vi "AddObject.vi"(8 "error in (no error)":errorcluster, 9 "OjbectName":string, 11 "Object2Add":refnum<class>) -> (0 "error out":errorcluster, 3 "ObjectOut":refnum<class>)   [LabVIEW 2021, in "Application.lvclass"]
uses:
  Application.lvclass
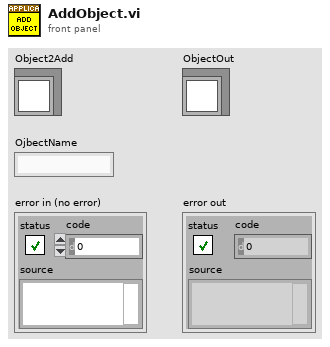
[diagram p1: front panel]
types:
  T1 = typedef "Application.lvclass/ObjectAttributes.ctl" = cluster{"Objects":variant, "BasePath":path, "Application":refnum<class "Application.lvclass">}
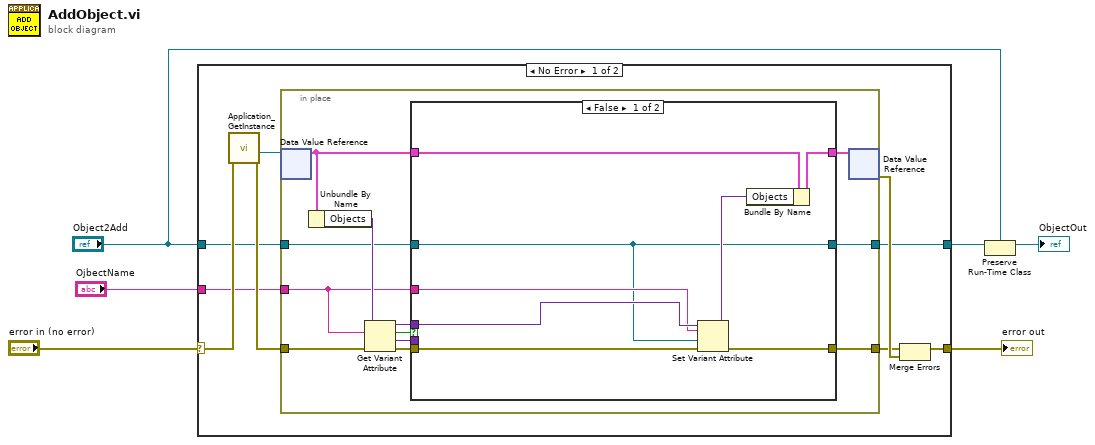
[diagram p0: block diagram]
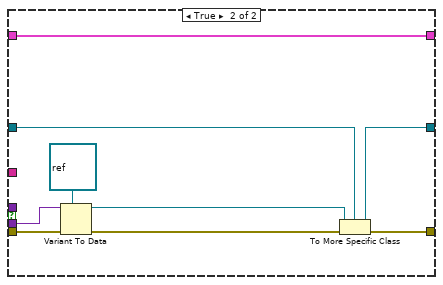
[diagram p2: hidden frame]
diagram:
  n1 = case shown="No Error" "error in (no error)" {
    selector: "error in (no error)" -> [w14 w45]
    tunnel: [w15 w45] -> w1
    tunnel: "OjbectName" -> [w10 _]
    tunnel: "Object2Add" -> [w9 _]
    tunnel: [w7 _] -> w5
    frame No Error {
      n2 = call "Application_GetInstance.vi"("error in"=w14) -> ("error out"=w11:errorcluster, "DVRRefOut"=w13:refnum<data-value>)  [unwired: 6 in, 3 out]
      n3 = in-place {
        in-place-border: w11 -> [w25]
        in-place-border: w10 -> [w17]
        in-place-border: w9 -> [w20]
        in-place-border: [w19] -> w8
        in-place-border: [w18] -> w7
        n4 = in-place-dvr #1(w13) -> (w26:T1)  [unwired: 1 out]
        n5 = Unbundle By Name(w26) -> ("Objects"=w24:variant)
        n6 = Get Variant Attribute(Variant=w24, name=w17, error in=w25) -> (duplicate Variant=w21:variant, found=w22:bool, value=w16:variant, error out=w23:errorcluster)  [unwired: 1 in]
        n7 = case shown="False" w22 {
          tunnel: [w32 w37] -> w27
          tunnel: w26 -> [w34 w37]
          tunnel: w23 -> [w28 w44]
          tunnel: w21 -> [w33 _]
          tunnel: w20 -> [w29 w40]
          tunnel: [w35 w42] -> w19
          tunnel: [w29 w38] -> w18
          tunnel: w17 -> [w31 _]
          tunnel: w16 -> [_ w36]
          frame False {
            n8 = Set Variant Attribute(Variant=w33, name=w31, value=w29, error in=w28) -> (Variant out=w30:variant, error out=w35:errorcluster)  [unwired: 1 out]
            n9 = Bundle By Name(cluster=w34, "Objects"=w30) -> (w32:T1)
          }
          frame True {
            n10 = Variant To Data(error in=w44, type=refnum<class> refnum ("Type"), Variant=w36) -> (data=w39:refnum<class>, error out=w43:errorcluster)
            n11 = To More Specific Class(target class=w40, reference=w39, error in=w43) -> (specific class reference=w38:refnum<class>, error out=w42:errorcluster)
          }
        }
        n12 = in-place-dvr #1(w27) -> (w12:errorcluster)  [unwired: 1 out]
      }
      n13 = Merge Errors(w8, w12) -> (w15:errorcluster)
    }
    frame Error {
    }
  }
  "error out" <- w1
  n14 = Preserve Run-Time Class(object in=w5, 2:"Object2Add") -> (object out=→"ObjectOut":refnum<class>)  [unwired: 1 in, 1 out]
